vi "Write session ref.vi"(8 "error in (no error)":errorcluster, 10 "session ref":refnum<k35>, 11 "Python Toolkit in":refnum<class "Python Toolkit.lvclass">) -> (0 "error out":errorcluster, 3 "Python Toolkit out":refnum<class "Python Toolkit.lvclass">)   [LabVIEW 2018, in "Python Toolkit.lvclass"]
uses:
  Python Toolkit.lvclass
  Python Toolkit.lvclass/Python Toolkit.ctl
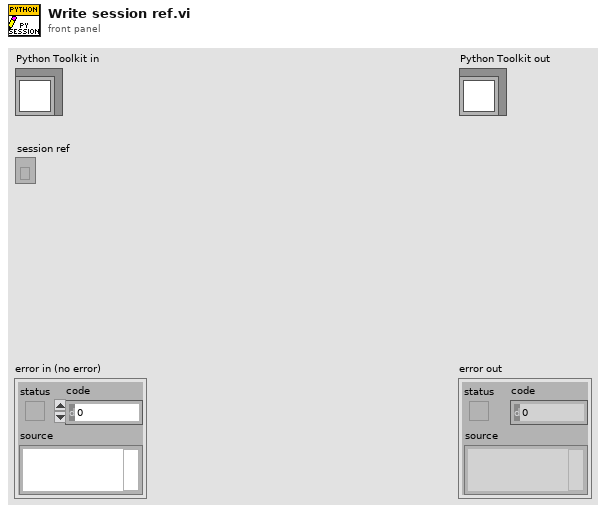
[diagram p1: front panel]
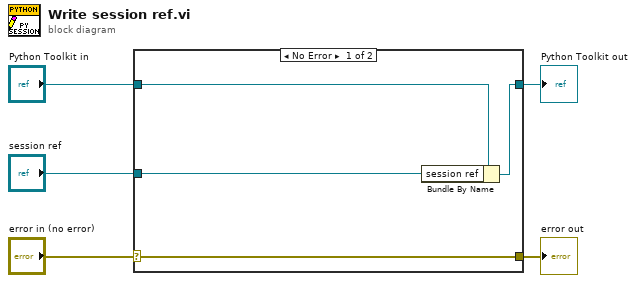
[diagram p0: block diagram]
diagram:
  n1 = case shown="No Error" "error in (no error)" {
    selector: "error in (no error)" -> [w9 w10]
    tunnel: [w9 w10] -> w4
    tunnel: [w7 w11] -> w2
    tunnel: "Python Toolkit in" -> [w8 w11]
    tunnel: "session ref" -> [w6 _]
    frame No Error {
      n2 = Bundle By Name(cluster=w8, "session ref"=w6) -> (w7:refnum<class "Python Toolkit.lvclass">)
    }
    frame Error {
    }
  }
  "error out" <- w4
  "Python Toolkit out" <- w2
